vi "Desnattor Interlock.vi"(11 "Seq1":enum16{"Seq_1", "Seq_2", "Seq_3", "Seq_4"}(ring)) -> (3 "Ready":bool)   [LabVIEW 2015]
uses:
  Galobal variable_TI.vi
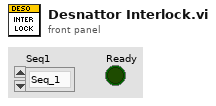
[diagram p1: front panel]
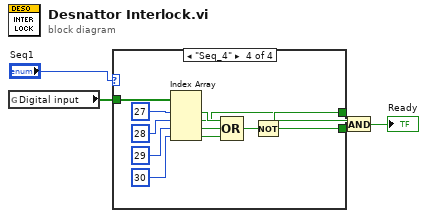
[diagram p0: block diagram]
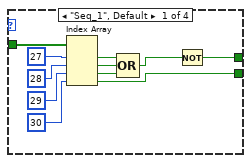
[diagram p2: hidden frame]
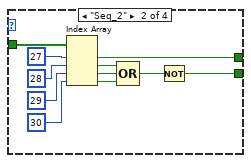
[diagram p3: hidden frame]
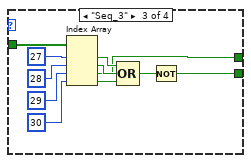
[diagram p4: hidden frame]
diagram:
  n1 = global read "Galobal variable_TI.vi" "Digital input"() -> (w2:bool[])
  n2 = case shown="\"Seq_4\"" "Seq1" {
    tunnel: w2 -> [w12 w21 w33 w43]
    tunnel: [w6 w19 w30 w41] -> w3
    tunnel: [w7 w17 w28 w39] -> w4
    frame "Seq_1", Default {
      n3 = Index Array(array=w12, index #1=27 ("index"), index #2=28 ("index"), index #3=29 ("index"), index #4=30 ("index")) -> (element #1=w11:bool, element #2=w10:bool, element #3=w9:bool, element #4=w7:bool)
      n4 = Compound Arithmetic op=OR(w11, w10, w9) -> (w8:bool)
      n5 = Not(x=w8) -> (.not. x?=w6:bool)
    }
    frame "Seq_2" {
      n6 = Index Array(array=w21, index #1=27 ("index"), index #2=28 ("index"), index #3=29 ("index"), index #4=30 ("index")) -> (element #1=w19:bool, element #2=w23:bool, element #3=w22:bool, element #4=w20:bool)
      n7 = Compound Arithmetic op=OR(w23, w22, w20) -> (w18:bool)
      n8 = Not(x=w18) -> (.not. x?=w17:bool)
    }
    frame "Seq_3" {
      n9 = Index Array(array=w33, index #1=27 ("index"), index #2=28 ("index"), index #3=29 ("index"), index #4=30 ("index")) -> (element #1=w32:bool, element #2=w31:bool, element #3=w30:bool, element #4=w34:bool)
      n10 = Compound Arithmetic op=OR(w32, w31, w34) -> (w29:bool)
      n11 = Not(x=w29) -> (.not. x?=w28:bool)
    }
    frame "Seq_4" {
      n12 = Index Array(array=w43, index #1=27 ("index"), index #2=28 ("index"), index #3=29 ("index"), index #4=30 ("index")) -> (element #1=w42:bool, element #2=w41:bool, element #3=w45:bool, element #4=w44:bool)
      n13 = Compound Arithmetic op=OR(w42, w45, w44) -> (w40:bool)
      n14 = Not(x=w40) -> (.not. x?=w39:bool)
    }
  }
  n15 = And(x=w3, y=w4) -> (x .and. y?=→"Ready":bool)
